vi "hidSPD Open Session.vi"(8 "error in (no error)":errorcluster, 11 "HidDevInfo":T7) -> (0 "error out":errorcluster, 3 "spdDevSession out":T1={"spdRef"=0, "connected"=FALSE, "spdName"="", "specification"={"diod case"=enum."default", "type"=enum."Unknown", "frequency"=enum."Unknown"}, "hidSPD.Controller"={"TSet"=0.0, "HV_bias"=0.0, "DDS_stb_code"=0}, "hidSPD.Sturtup Values"={"TSet"=0.0, "HV_bias"=0.0, "DDS_stb_code"=0}} {"hidSPD.Sturtup Values"."HV_bias" format="%#_6p, V"; "hidSPD.Sturtup Values"."TSet" format="%#_6p, DegC"; "hidSPD.Controller"."HV_bias" format="%#_6p, V"; "hidSPD.Controller"."TSet" format="%#_6p, DegC"})   [LabVIEW 2018, in "hidSPDLibForLabView.lvlib"]
uses:
  hidSPDLibForLabView.lvlib
  hidSPD Controls/hidSPD HidDevInfo.ctl
  hidSPD Controls/hidSPD Device Session.ctl
  hidSPD Controls/hidSPD.SPD specification.ctl
  hidSPD Controls/hidSPD SPD Diod Case.ctl
  hidSPD Controls/hidSPD SPD Type.ctl
  hidSPD Controls/hidSPD.STB Frequency.ctl
  hidSPD Controls/hidSPD Controller.ctl
  <vilib>/Utility/error.llb/Error Cluster From Error Code.vi
  <vilib>/ErrorRing/Error Ring.xnode
  hidSPD DLL files/libSPD.dll
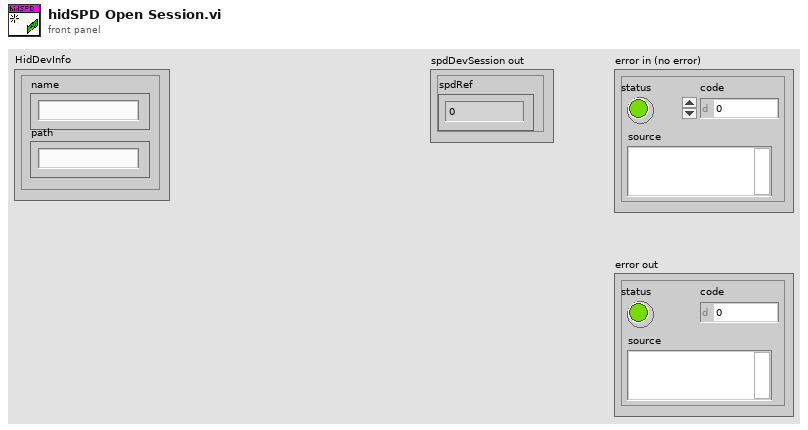
[diagram p1: front panel]
types:
  T1 = typedef "hidSPDLibForLabView.lvlib/hidSPD Device Session.ctl" = cluster{"spdRef":u64, "connected":bool, "spdName":string, "specification":T2, "hidSPD.Controller":T6, "hidSPD.Sturtup Values":T6}
  T2 = typedef "hidSPDLibForLabView.lvlib/hidSPD.SPD specification.ctl" = cluster{"diod case":T3, "type":T4, "frequency":T5}
  T3 = typedef "hidSPDLibForLabView.lvlib/hidSPD SPD Diod Case.ctl" = enum16{"Unknown", "default", "butterfly"}
  T4 = typedef "hidSPDLibForLabView.lvlib/hidSPD SPD Type.ctl" = enum16{"Unknown", "Free Run", "Gate"}
  T5 = typedef "hidSPDLibForLabView.lvlib/hidSPD.STB Frequency.ctl" = enum16{"Unknown", "312", "1250"}
  T6 = typedef "hidSPDLibForLabView.lvlib/hidSPD Controller.ctl" = cluster{"TSet":sgl, "HV_bias":sgl, "DDS_stb_code":u16}
  T7 = typedef "hidSPDLibForLabView.lvlib/hidSPD HidDevInfo.ctl" = cluster{"name":string, "path":string}
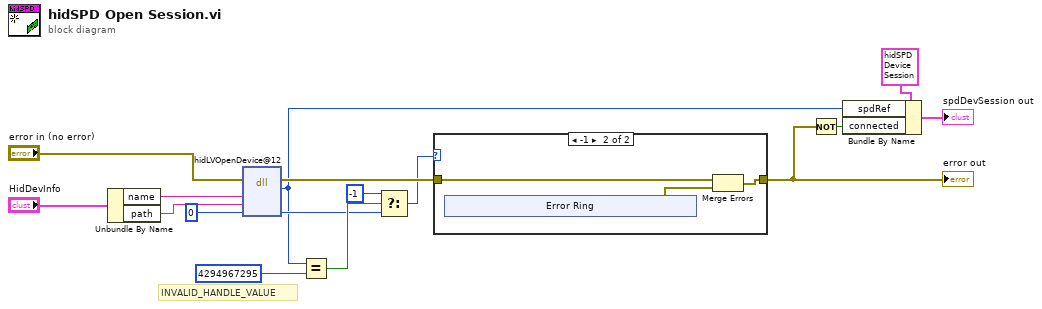
[diagram p0: block diagram]
diagram:
  # "INVALID_HANDLE_VALUE"
  n1 = Unbundle By Name("HidDevInfo") -> ("name"=w12:string, "path"=w11:string)
  n2 = dll-call lib="D:/NextCloud/SPD stand/Automative SPD Measurements/Automative SPD Stand/Instruments/SPD HID Interface/hidSPDLibForLabView/hidSPD DLL files/libSPD.dll" fn="hidLVOpenDevice@12"(error in="error in (no error)", "deviceName"=w12, "devicePath"=w11, "errorCode"=0 ("deguflength")) -> (error out=w15:errorcluster, "spdDevHandle"=w4:u64, "errorCode"=w8:i32)  [unwired: 4 in, 1 out]
  n3 = Equal?(x=w4, y=u64 4294967295) -> (x = y?=w9:bool)
  n4 = Select(t=-1, s=w9, f=w8) -> (s? t:f=w6:i32)
  n5 = case shown="-1" w6 {
    tunnel: w15 -> [w17 w20]
    tunnel: [w17 w18] -> w1
    frame 0, Default {
    }
    frame -1 {
      n6 = xnode "Error Ring"() -> ("error out"=w19:errorcluster)
      n7 = Merge Errors(w20, w19) -> (w18:errorcluster)
    }
  }
  "error out" <- w1
  n8 = Not(x=w1) -> (.not. x?=w2:bool)
  n9 = Bundle By Name(cluster=T1 {"spdRef"=0, "connected"=FALSE, "spdName"="", "specification"={"diod case"=enum."default", "type"=enum."Unknown", "frequency"=enum."Unknown"}, "hidSPD.Controller"={"TSet"=0.0, "HV_bias"=0.0, "DDS_stb_code"=0}, "hidSPD.Sturtup Values"={"TSet"=0.0, "HV_bias"=0.0, "DDS_stb_code"=0}} ("spdDeviceSession"), "spdRef"=w4, "connected"=w2) -> (→"spdDevSession out":T1)
